vi "FTW-Subscription-Destroy.vi"(0 "FTW-Subscription In":refnum<class "FTW-Subscription.lvclass">, 11 "error in":errorcluster) -> (15 "error out":errorcluster)   [LabVIEW 2013, in "FTW-Subscription.lvclass"]
uses:
  FTW-Subscription.lvclass
  FTW-Subscription.lvclass/FTW-Subscription.ctl
  Endpoint/FTW-Endpoint.lvclass
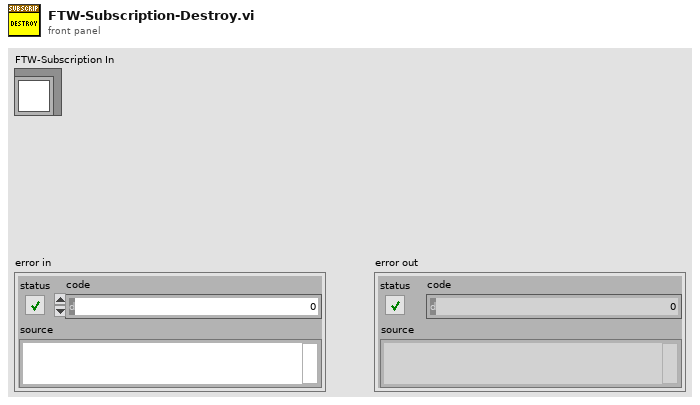
[diagram p1: front panel]
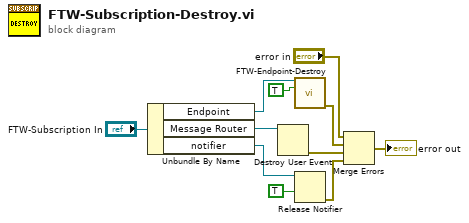
[diagram p0: block diagram]
diagram:
  n1 = Unbundle By Name("FTW-Subscription In") -> ("Endpoint"=w7:refnum<class "FTW-Endpoint.lvclass">, "Message Router"=w8:refnum<user-event>, "notifier"=w3:refnum<notifier>)
  n2 = Destroy User Event(user event=w8) -> (error out=w5:errorcluster)  [unwired: 1 in]
  n3 = call-dynamic "FTW-Endpoint-Destroy.vi"("FTW Endpoint"=w7, "Force Destroy"=TRUE) -> ("error out"=w6:errorcluster)  [unwired: 13 in]
  n4 = Release Notifier(notifier=w3, force destroy? (F)=TRUE) -> (error out=w1:errorcluster)  [unwired: 1 in, 2 out]
  n5 = Merge Errors("error in", w6, w5, w1) -> (→"error out":errorcluster)
